vi "MQTT_PubAck_Read.vi"(8 "error in (no error)":errorcluster, 11 "connection ID":refnum<k5>) -> (0 "error out":errorcluster, 2 "Message ID":u16=10 format="%x", 3 "connection ID out":refnum<k5>)   [LabVIEW 2025, in "DAQIO MQTT.lvlib"]
doc: "© 2015 - daq.io, LLC - Peter Adelhardt"
uses:
  DAQIO MQTT.lvlib
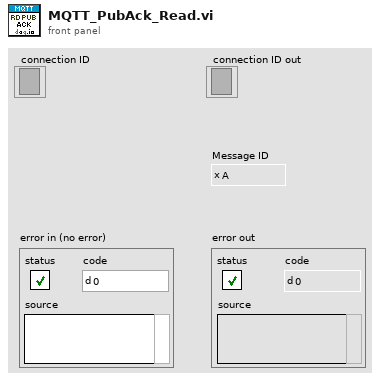
[diagram p1: front panel]
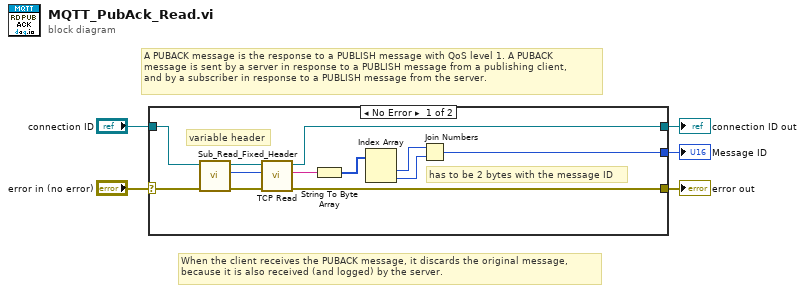
[diagram p0: block diagram]
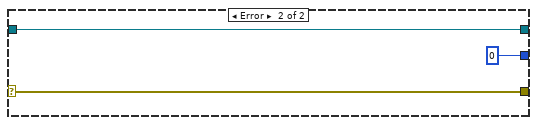
[diagram p2: hidden frame]
diagram:
  # "When the client receives the PUBACK message, it discards the original message,\nbecause it is also received (and logged) by the server."
  # "A PUBACK message is the response to a PUBLISH message with QoS level 1. A PUBACK\nmessage is sent by a server in response to a PUBLISH message from a publishing client,\nand by a subscriber in response to a PUBLISH message from the server."
  n1 = case shown="No Error" "error in (no error)" {
    selector: "error in (no error)" -> [w17 w20]
    tunnel: [w11 w20] -> w4
    tunnel: "connection ID" -> [w8 w18]
    tunnel: [w7 w18] -> w2
    tunnel: [w6 u16 0] -> w1
    frame No Error {
      # "has to be 2 bytes with the message ID"
      # "variable header"
      n2 = call "Sub_Read_Fixed_Header.vi"("error in (no error)"=w17, "connection ID"=w8) -> ("error out"=w15:errorcluster, "Remaining Length"=w16:u32, "connection ID out"=w14:refnum<k5>)  [unwired: 3 in, 4 out]
      n3 = call "TCP Read.vi"("error in (no error)"=w15, "bytes to read"=w16, "connection ID"=w14) -> ("error out"=w11:errorcluster, "data out"=w13:string, "connection ID out"=w7:refnum<k5>)  [unwired: 6 in]
      n4 = String To Byte Array(string=w13) -> (unsigned byte array=w12:u8[])
      n5 = Index Array(array=w12) -> (element #1=w9:u8, element #2=w10:u8)  [unwired: 2 in]
      n6 = Join Numbers(hi=w9, lo=w10) -> ((hi.lo)=w6:u16)
    }
    frame Error {
    }
  }
  "error out" <- w4
  "Message ID" <- w1
  "connection ID out" <- w2
